vi "parse.vi"(8 "error in (no error)":errorcluster, 10 "DynamicFrameParser":refnum<class "DynamicFrameParser.lvclass">, 11 "MTILC in":refnum<class "MTILC.lvclass">) -> (0 "error out":errorcluster, 2 "ParseSuccessful":bool, 3 "MTILC out":refnum<class "MTILC.lvclass">)   [LabVIEW 2016, in "RTMTILC.lvlib" / "MTILC.lvclass"]
uses:
  MTILC.lvclass
  Common_RT_Modbus/DynamicFrameParser/DynamicFrameParser.lvclass
  Common_RT_ILC/ILC/ILC.lvclass
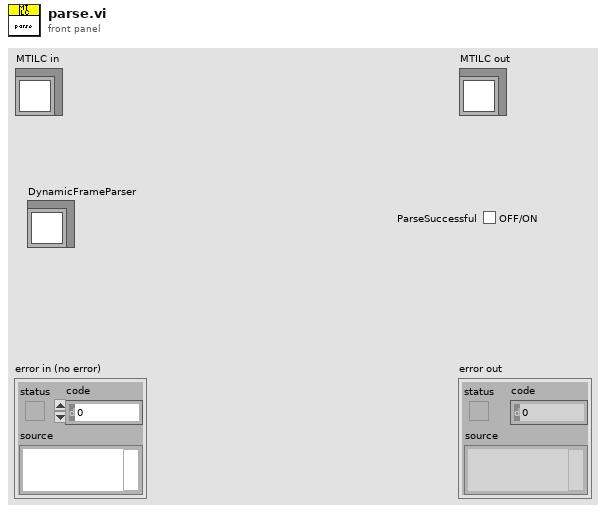
[diagram p1: front panel]
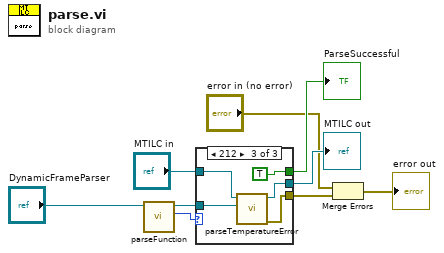
[diagram p0: block diagram]
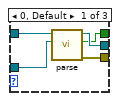
[diagram p2: hidden frame]
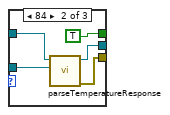
[diagram p3: hidden frame]
diagram:
  n1 = call "parseFunction.vi"("FrameParser in"="DynamicFrameParser") -> ("Function"=w8:u8, "FrameParser out"=w1:refnum<class "DynamicFrameParser.lvclass">)  [unwired: 8 in, 1 out]
  n2 = case shown="212" w8 {
    tunnel: "MTILC in" -> [w14 w19 w24]
    tunnel: [w13 w18 w23] -> w6
    tunnel: [w12 TRUE ("ParseSuccessful") TRUE ("ParseSuccessful")] -> w5
    tunnel: [w11 w16 w21] -> w4
    tunnel: w1 -> [w10 w15 w20]
    frame 0, Default {
      n3 = call-parent "parse.vi"("DynamicFrameParser"=w10, "ILC in"=w14) -> ("error out"=w11:errorcluster, "ParseSuccessful"=w12:bool, "ILC out"=w13:refnum<class "MTILC.lvclass">)  [unwired: 7 in]
    }
    frame 84 {
      n4 = call "parseTemperatureResponse.vi"("DynamicFrameParser"=w15, "MTILC in"=w19) -> ("error out"=w16:errorcluster, "MTILC out"=w18:refnum<class "MTILC.lvclass">)  [unwired: 8 in]
    }
    frame 212 {
      n5 = call "parseTemperatureError.vi"("DynamicFrameParser"=w20, "MTILC in"=w24) -> ("error out"=w21:errorcluster, "MTILC out"=w23:refnum<class "MTILC.lvclass">)  [unwired: 8 in]
    }
  }
  "MTILC out" <- w6
  "ParseSuccessful" <- w5
  n6 = Merge Errors("error in (no error)", w4) -> (→"error out":errorcluster)
